vi "PLC控制测试.vi"() -> ()   [LabVIEW 2014]
uses:
  <vilib>/Instr/_visa.llb/VISA Configure Serial Port (Instr).vi
  R/manifest.vi
panel:
  out "复位":bool
  out "体验结束":bool
  out "开始体验":bool
  out "开门":bool
  out "急停":bool
  out "2进制字符串 2":string
  in  "急停":bool
  in  "复位":bool
  in  "结束体验":bool
  in  "开始体验":bool
  in  "开门":bool
  out "read buffer":string
  out "error IO":errorcluster
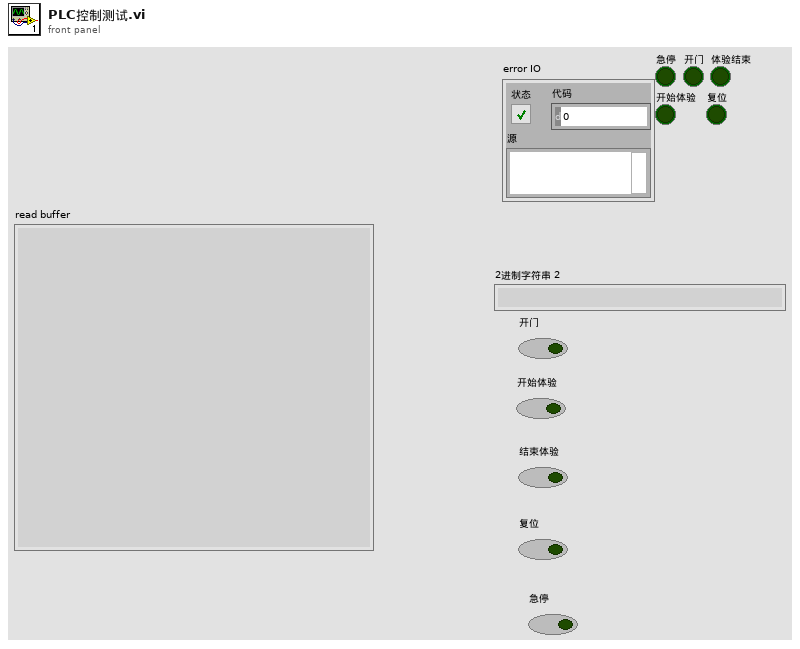
[diagram p1: front panel]
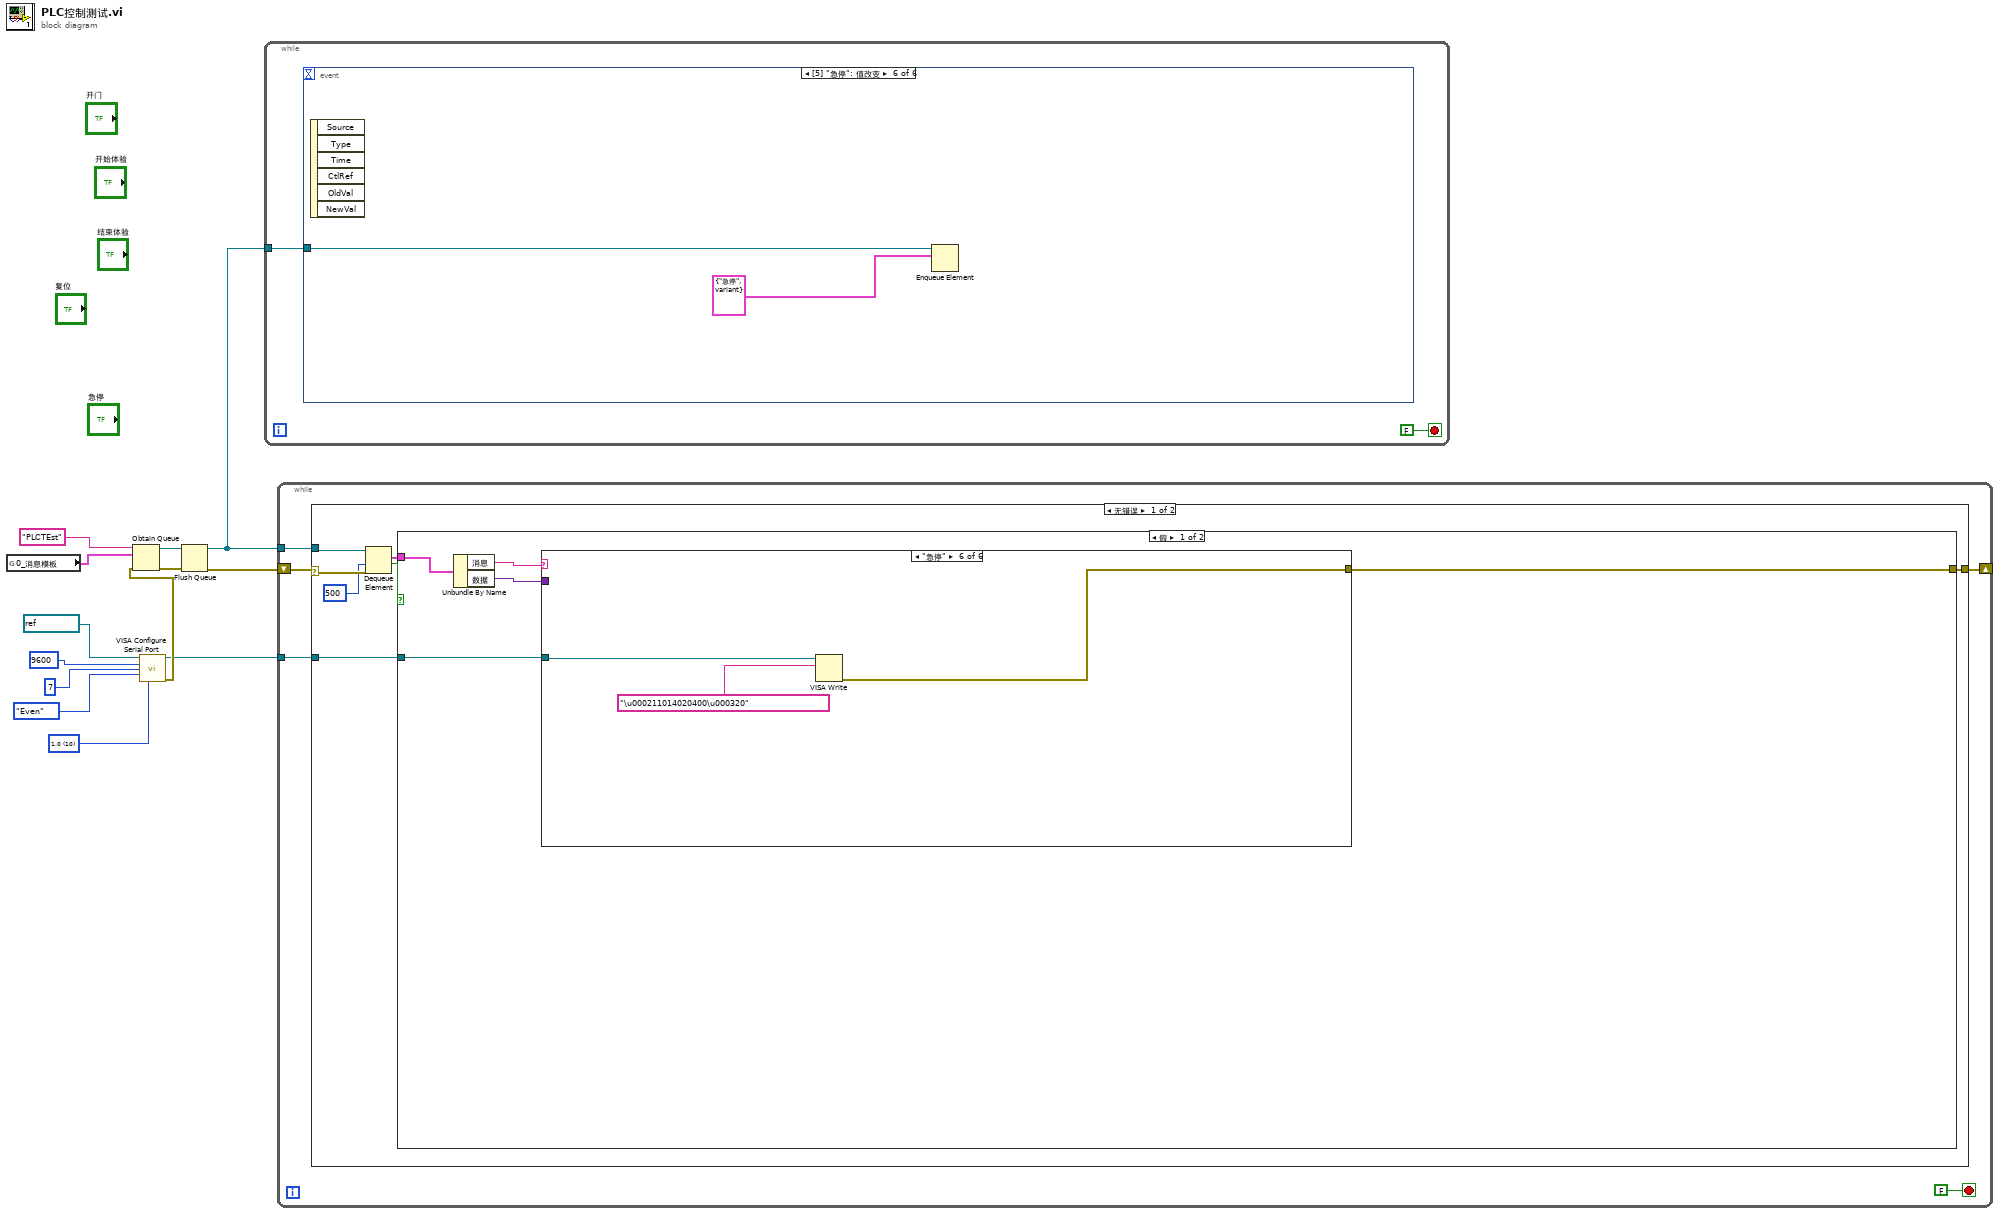
[diagram p0: block diagram]
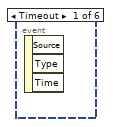
[diagram p2: hidden frame]
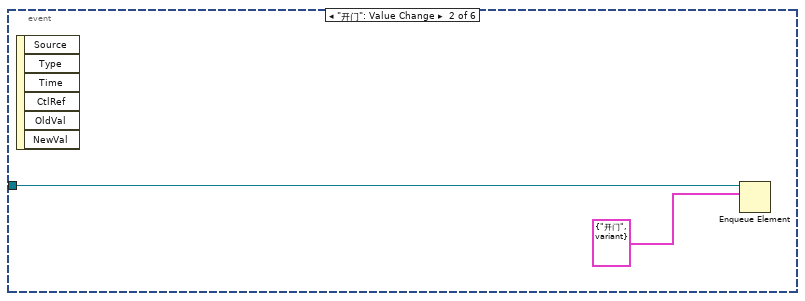
[diagram p3: hidden frame]
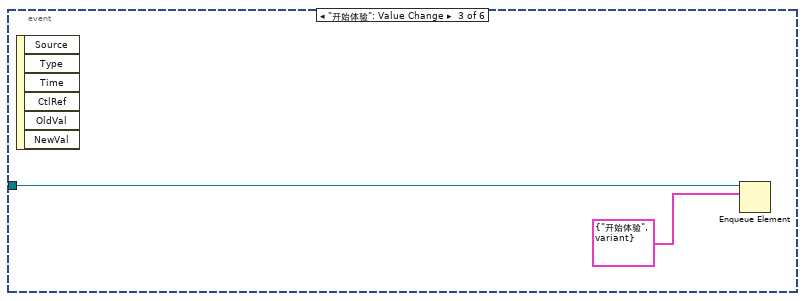
[diagram p4: hidden frame]
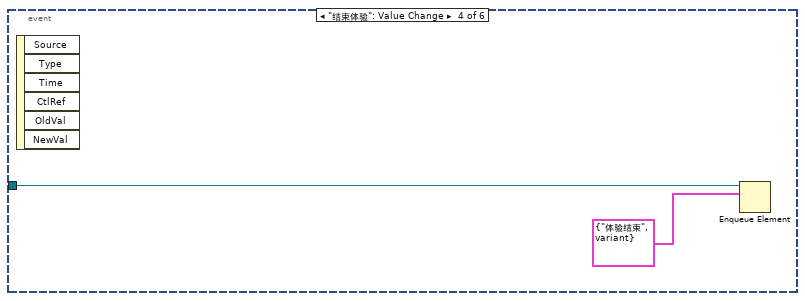
[diagram p5: hidden frame]
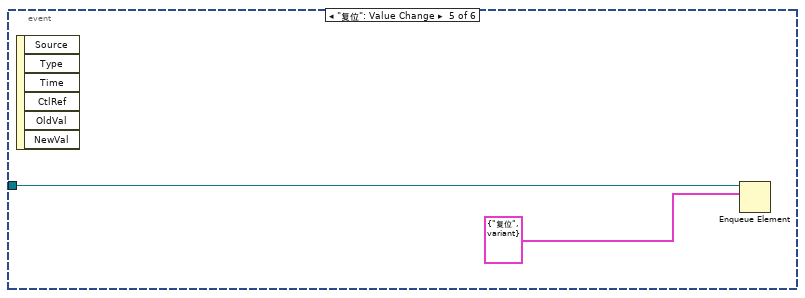
[diagram p6: hidden frame]
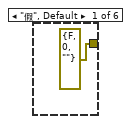
[diagram p7: hidden frame]
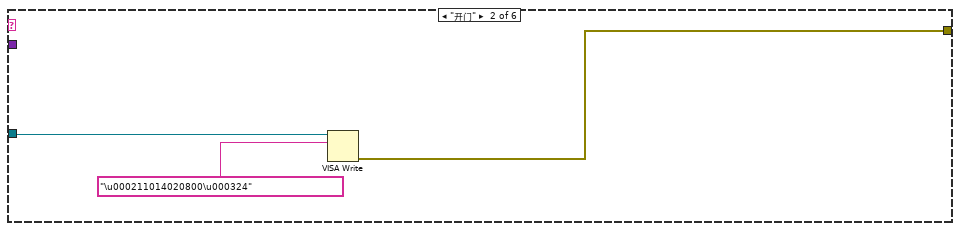
[diagram p8: hidden frame]
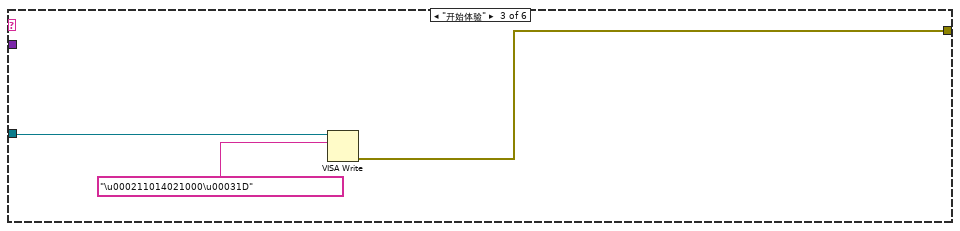
[diagram p9: hidden frame]
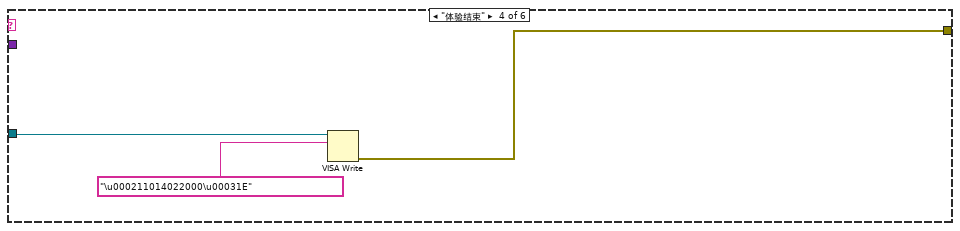
[diagram p10: hidden frame]
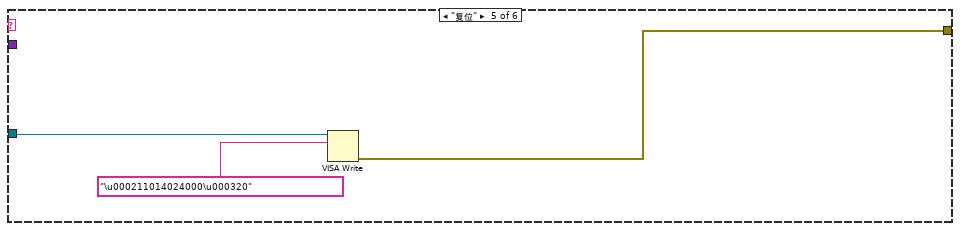
[diagram p11: hidden frame]
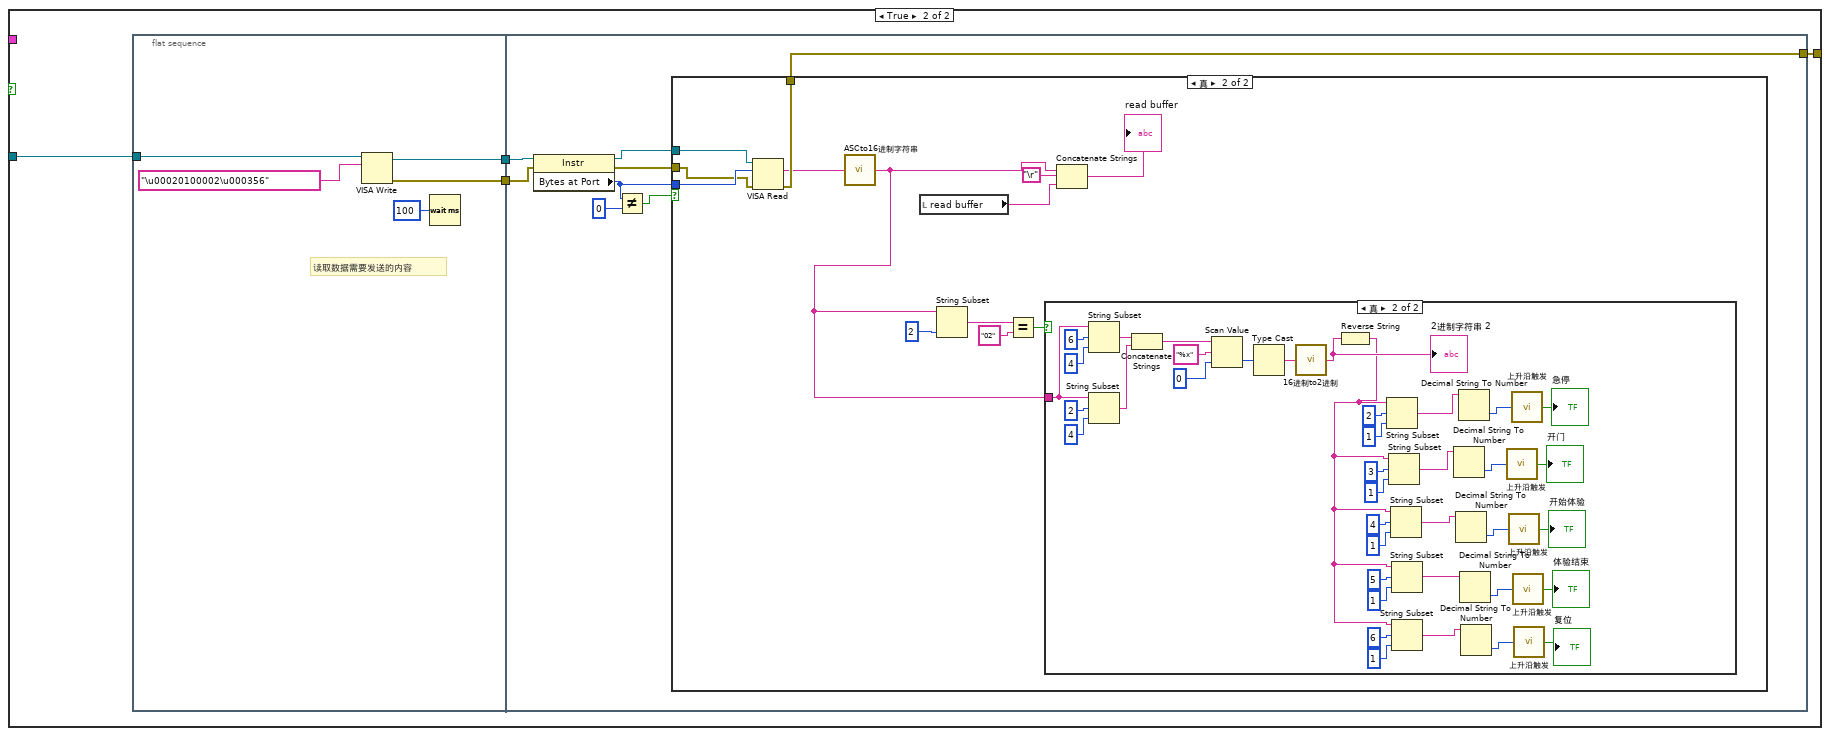
[diagram p12: hidden frame]
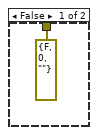
[diagram p13: hidden frame]
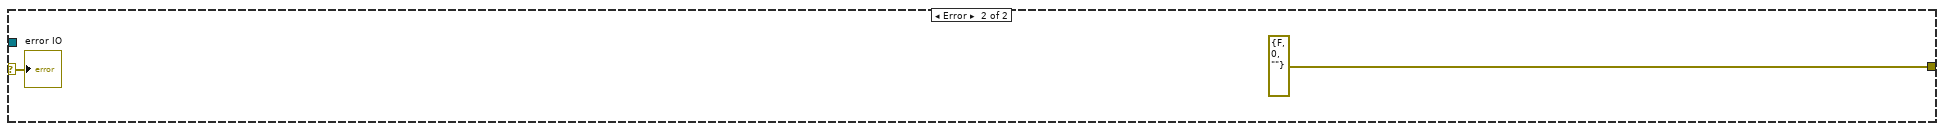
[diagram p15: hidden frame]
diagram:
  w10 = u16 10 items=["1.0"=10, "1.5"=15, "2.0"=20] ("stop bits (10: 1 bit)")
  n1 = global read "manifest.vi" "0_消息模板"() -> (w8:cluster{"消息":string, "数据":variant})
  n2 = call-poly "VISA Configure Serial Port"("VISA resource name"=refnum<visa-resource-name> "COM5", "baud rate (9600)"=u32 9600, "data bits (8)"=u16 7, "parity (0:none)"=enum16{"None", "Odd", "Even", "Mark", "Space"}."Even", "stop bits (10: 1 bit)"=w10) -> ("VISA resource name out"=w3:refnum<visa-resource-name>, "error out"=w4:errorcluster)  [unwired: 9 in]
  n3 = Obtain Queue(name (unnamed)="PLCTEst" ("名称（未命名）"), element data type=w8, error in (no error)=w4) -> (queue out=w7:refnum<queue>, error out=w6:errorcluster)  [unwired: 2 in, 1 out]
  n4 = Flush Queue(queue=w7, error in (no error)=w6) -> (queue out=w1:refnum<queue>, error out=w5:errorcluster)  [unwired: 1 out]
  n5 = while {
    tunnel: w1 -> [w14]
    stop <- FALSE stop-if-true
    n6 = event shown="[5] \"急停\": 值改变" {
      selector: _ -> [_ _ _ _ _ _]
      dyn-events: _ -> [_ _ _ _ _ _]
      timeout: _ -> [_ _ _ _ _ _]
      tunnel: w14 -> [_ w17 w19 w21 w23 w25]
      event Timeout {
        n7 = event-data() -> ()  [unwired: 1 in, 3 out]
      }
      event "开门": Value Change {
        n8 = event-data() -> ()  [unwired: 1 in, 6 out]
        n9 = Enqueue Element(queue=w17, element=cluster{"消息":string, "数据":variant} {"消息"="开门", "数据"=variant} ("元素")) -> ()  [unwired: 2 in, 3 out]
      }
      event "开始体验": Value Change {
        n10 = event-data() -> ()  [unwired: 1 in, 6 out]
        n11 = Enqueue Element(queue=w19, element=cluster{"消息":string, "数据":variant} {"消息"="开始体验", "数据"=variant} ("元素")) -> ()  [unwired: 2 in, 3 out]
      }
      event "结束体验": Value Change {
        n12 = event-data() -> ()  [unwired: 1 in, 6 out]
        n13 = Enqueue Element(queue=w21, element=cluster{"消息":string, "数据":variant} {"消息"="体验结束", "数据"=variant} ("元素")) -> ()  [unwired: 2 in, 3 out]
      }
      event "复位": Value Change {
        n14 = event-data() -> ()  [unwired: 1 in, 6 out]
        n15 = Enqueue Element(queue=w23, element=cluster{"消息":string, "数据":variant} {"消息"="复位", "数据"=variant} ("元素")) -> ()  [unwired: 2 in, 3 out]
      }
      event "急停": Value Change {
        n16 = event-data() -> ()  [unwired: 1 in, 6 out]
        n17 = Enqueue Element(queue=w25, element=cluster{"消息":string, "数据":variant} {"消息"="急停", "数据"=variant} ("元素")) -> ()  [unwired: 2 in, 3 out]
      }
    }
  }
  n18 = while {
    tunnel: w1 -> [w28]
    shift-right: [w26] -> _
    shift-left: w5 -> [w29]
    tunnel: w3 -> [w27]
    stop <- FALSE stop-if-true
    n19 = case shown="无错误" w29 {
      selector: w29 -> [w36 w130]
      tunnel: w28 -> [w37 _]
      tunnel: w27 -> [w32 _]
      tunnel: [w31 errorcluster {"status"=FALSE, "code"=0, "source"=""} ("error out")] -> w26
      frame No Error {
        n20 = Dequeue Element(queue=w37, timeout in ms (-1)=500 ("超时毫秒(-1)"), error in (no error)=w36) -> (element=w35:cluster{"消息":string, "数据":variant}, timed out?=w33:bool)  [unwired: 2 out]
        n21 = case shown="假" w33 {
          tunnel: w35 -> [w42 _]
          tunnel: w32 -> [w39 w62]
          tunnel: [w38 w59] -> w31
          frame False {
            n22 = Unbundle By Name(w42) -> ("消息"=w41:string, "数据"=w40:variant)
            n23 = case shown="\"急停\"" w41 {
              tunnel: w40 -> [_ _ _ _ _ _]
              tunnel: w39 -> [_ w46 w49 w52 w55 w58]
              tunnel: [errorcluster {"status"=FALSE, "code"=0, "source"=""} ("error out") w44 w47 w50 w53 w56] -> w38
              frame "假", Default {
              }
              frame "开门" {
                n24 = VISA Write(VISA resource name=w46, write buffer="\u000211014020800\u000324" ("写入缓冲区")) -> (error out=w44:errorcluster)  [unwired: 1 in, 2 out]
              }
              frame "开始体验" {
                n25 = VISA Write(VISA resource name=w49, write buffer="\u000211014021000\u00031D" ("写入缓冲区")) -> (error out=w47:errorcluster)  [unwired: 1 in, 2 out]
              }
              frame "体验结束" {
                n26 = VISA Write(VISA resource name=w52, write buffer="\u000211014022000\u00031E" ("写入缓冲区")) -> (error out=w50:errorcluster)  [unwired: 1 in, 2 out]
              }
              frame "复位" {
                n27 = VISA Write(VISA resource name=w55, write buffer="\u000211014024000\u000320" ("写入缓冲区")) -> (error out=w53:errorcluster)  [unwired: 1 in, 2 out]
              }
              frame "急停" {
                n28 = VISA Write(VISA resource name=w58, write buffer="\u000211014020400\u000320" ("写入缓冲区")) -> (error out=w56:errorcluster)  [unwired: 1 in, 2 out]
              }
            }
          }
          frame True {
            n29 = flat-sequence {
              tunnel: w62 -> [w67]
              tunnel: [w64] -> w61
              tunnel: [w63] -> w60
              tunnel: w61 -> [w73]
              tunnel: w60 -> [w72]
              tunnel: [w68] -> w59
              frame #0 {
                # "读取数据需要发送的内容"
                n30 = VISA Write(VISA resource name=w67, write buffer="\u00020100002\u000356" ("写入缓冲区")) -> (VISA resource name out=w64:refnum<visa-resource-name>, error out=w63:errorcluster)  [unwired: 1 in, 1 out]
                n31 = Wait (ms)(milliseconds to wait=u32 100 ("等待时间（毫秒）")) -> ()  [unwired: 1 out]
              }
              frame #1 {
                n32 = property class="Instr"(reference=w73, error in=w72) -> (reference out=w70:refnum<visa-resource-name>, error out=w71:errorcluster, "Bytes at Port"=w69:u32)
                n33 = Not Equal?(x=w69, y=u32 0) -> (x != y?=w74:bool)
                n34 = case shown="真" w74 {
                  tunnel: w71 -> [_ w87]
                  tunnel: w70 -> [_ w88]
                  tunnel: w69 -> [_ w89]
                  tunnel: [errorcluster {"status"=FALSE, "code"=0, "source"=""} ("error out") w86] -> w68
                  frame False {
                  }
                  frame True {
                    n35 = VISA Read(VISA resource name=w88, byte count=w89, error in (no error)=w87) -> (read buffer=w85:string, error out=w86:errorcluster)  [unwired: 2 out]
                    n36 = call "ASCto16进制字符串.vi"("ASC"=w85) -> ("16进制字符串"=w77:string)
                    n37 = local read "read buffer"() -> (w83:string)
                    n38 = String Subset(string=w77, length (rest)=2 ("长度（剩余）")) -> (substring=w80:string)  [unwired: 1 in]
                    n39 = Equal?(x=w80, y="02") -> (x = y?=w78:bool)
                    n40 = case shown="真" w78 {
                      tunnel: w77 -> [_ w124]
                      frame False {
                      }
                      frame True {
                        n41 = String Subset(string=w124, offset (0)=6 ("偏移量(0)"), length (rest)=4 ("长度（剩余）")) -> (substring=w123:string)
                        n42 = String Subset(string=w124, offset (0)=2 ("偏移量(0)"), length (rest)=4 ("长度（剩余）")) -> (substring=w122:string)
                        n43 = Concatenate Strings(w123, w122) -> (w121:string)
                        n44 = Scan Value(string=w121, format string="%x", default (0 dbl)=0) -> (value=w118:i32)  [unwired: 1 out]
                        n45 = Type Cast(x=w118) -> (*(type *) &x=w117:string)  [unwired: 1 in]
                        n46 = call "16进制to2进制.vi"("16进制字符串"=w117) -> ("2进制字符串"=w106:string)
                        "2进制字符串 2" <- w106
                        n47 = Reverse String(1:w106) -> (0:w105:string)
                        n48 = String Subset(string=w105, offset (0)=2 ("偏移量(0)"), length (rest)=1 ("长度（剩余）")) -> (substring=w104:string)
                        n49 = String Subset(string=w105, offset (0)=3 ("偏移量(0)"), length (rest)=1 ("长度（剩余）")) -> (substring=w98:string)
                        n50 = String Subset(string=w105, offset (0)=4 ("偏移量(0)"), length (rest)=1 ("长度（剩余）")) -> (substring=w97:string)
                        n51 = String Subset(string=w105, offset (0)=5 ("偏移量(0)"), length (rest)=1 ("长度（剩余）")) -> (substring=w96:string)
                        n52 = String Subset(string=w105, offset (0)=6 ("偏移量(0)"), length (rest)=1 ("长度（剩余）")) -> (substring=w95:string)
                        n53 = Decimal String To Number(string=w98) -> (number=w102:i32)  [unwired: 2 in, 1 out]
                        n54 = Decimal String To Number(string=w97) -> (number=w101:i32)  [unwired: 2 in, 1 out]
                        n55 = Decimal String To Number(string=w104) -> (number=w103:i32)  [unwired: 2 in, 1 out]
                        n56 = Decimal String To Number(string=w96) -> (number=w100:i32)  [unwired: 2 in, 1 out]
                        n57 = Decimal String To Number(string=w95) -> (number=w99:i32)  [unwired: 2 in, 1 out]
                        n58 = call "上升沿触发.vi"("信号输入"=w102) -> ("x与y?"=→"开门":bool)
                        n59 = call "上升沿触发.vi"("信号输入"=w101) -> ("x与y?"=→"开始体验":bool)
                        n60 = call "上升沿触发.vi"("信号输入"=w103) -> ("x与y?"=→"急停":bool)
                        n61 = call "上升沿触发.vi"("信号输入"=w100) -> ("x与y?"=→"体验结束":bool)
                        n62 = call "上升沿触发.vi"("信号输入"=w99) -> ("x与y?"=→"复位":bool)
                      }
                    }
                    n63 = Concatenate Strings(w77, "\r", w83) -> (→"read buffer":string)
                  }
                }
              }
            }
          }
        }
      }
      frame Error {
        "error IO" <- w130
      }
    }
  }
